vi "RemoveSpces.vi"(7 "input string":string) -> (8 "result string":string)   [LabVIEW 2023]
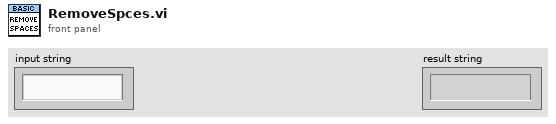
[diagram p1: front panel]
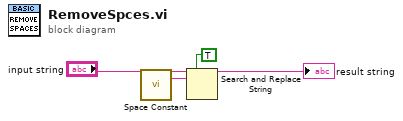
[diagram p0: block diagram]
diagram:
  n1 = call <vilib>:"Space Constant.vi"() -> ("String"=w4:string)
  n2 = Search and Replace String(replace all?=TRUE ("replace all? (F)"), input string="input string", search string=w4) -> (result string=→"result string":string)  [unwired: 5 in, 3 out]
